vi "gettangentjob.vi"(0 "sample port":refnum<visa-resource-name>[](array[refnum]), 2 "sample sn":string[](array[string])) -> (6 "tangent":dbl[](array[numeric]), 7 "Array":bool[](array[boolean]))   [LabVIEW 2012]
uses:
  globalstatus.vi
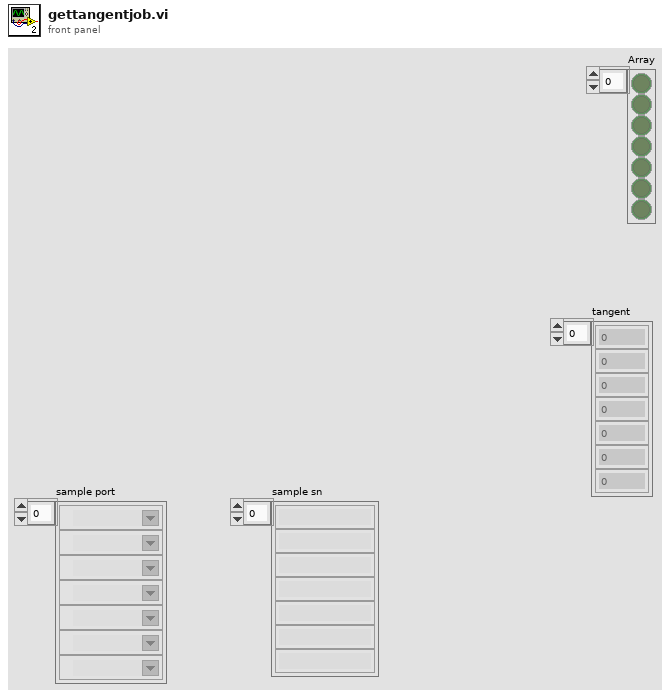
[diagram p1: front panel]
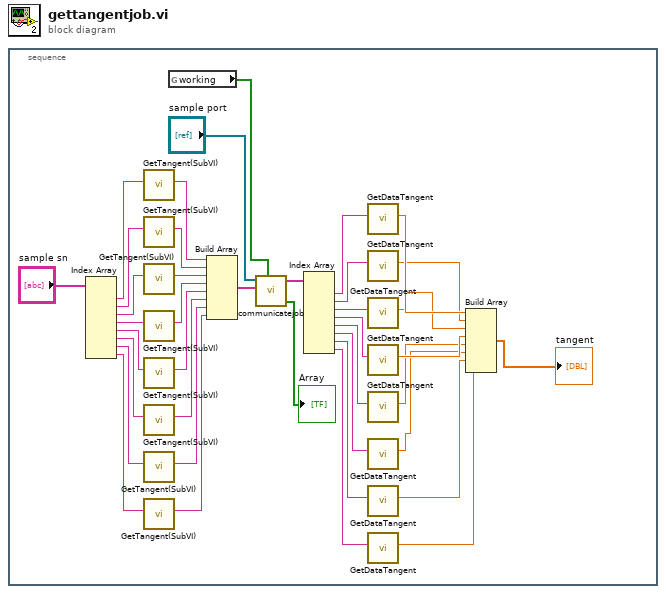
[diagram p0: block diagram]
diagram:
  n1 = stacked-sequence {
    frame #0 {
      n2 = Index Array(array="sample sn") -> (element #1=w38:string, element #2=w37:string, element #3=w36:string, element #4=w35:string, element #5=w34:string, element #6=w33:string, element #7=w32:string, element #8=w31:string)  [unwired: 8 in]
      n3 = call "GetTangent(SubVI).vi"("sn"=w38) -> ("output frame"=w28:string)  [unwired: 10 in]
      n4 = call "GetTangent(SubVI).vi"("sn"=w37) -> ("output frame"=w27:string)  [unwired: 10 in]
      n5 = call "GetTangent(SubVI).vi"("sn"=w36) -> ("output frame"=w26:string)  [unwired: 10 in]
      n6 = call "GetTangent(SubVI).vi"("sn"=w35) -> ("output frame"=w25:string)  [unwired: 10 in]
      n7 = call "GetTangent(SubVI).vi"("sn"=w34) -> ("output frame"=w24:string)  [unwired: 10 in]
      n8 = call "GetTangent(SubVI).vi"("sn"=w33) -> ("output frame"=w23:string)  [unwired: 10 in]
      n9 = call "GetTangent(SubVI).vi"("sn"=w32) -> ("output frame"=w22:string)  [unwired: 10 in]
      n10 = call "GetTangent(SubVI).vi"("sn"=w31) -> ("output frame"=w21:string)  [unwired: 10 in]
      n11 = global read "globalstatus.vi" "working"() -> (w29:bool[])
      n12 = Build Array(w28, w27, w26, w25, w24, w23, w22, w21) -> (w20:string[])
      n13 = call "communicatejob.vi"("sample port"="sample port", "condition"=w29, "send command"=w20) -> ("receive data"=w18:string[], "receive result"=→"Array":bool[])  [unwired: 2 in, 2 out]
      n14 = Index Array(array=w18) -> (element #1=w17:string, element #2=w16:string, element #3=w15:string, element #4=w14:string, element #5=w13:string, element #6=w12:string, element #7=w11:string, element #8=w10:string)  [unwired: 8 in]
      n15 = call "GetDataTangent.vi"("input data"=w17) -> ("tangent"=w9:dbl)  [unwired: 10 in]
      n16 = call "GetDataTangent.vi"("input data"=w16) -> ("tangent"=w8:dbl)  [unwired: 10 in]
      n17 = call "GetDataTangent.vi"("input data"=w15) -> ("tangent"=w7:dbl)  [unwired: 10 in]
      n18 = call "GetDataTangent.vi"("input data"=w14) -> ("tangent"=w6:dbl)  [unwired: 10 in]
      n19 = call "GetDataTangent.vi"("input data"=w13) -> ("tangent"=w5:dbl)  [unwired: 10 in]
      n20 = call "GetDataTangent.vi"("input data"=w12) -> ("tangent"=w4:dbl)  [unwired: 10 in]
      n21 = call "GetDataTangent.vi"("input data"=w11) -> ("tangent"=w3:dbl)  [unwired: 10 in]
      n22 = call "GetDataTangent.vi"("input data"=w10) -> ("tangent"=w2:dbl)  [unwired: 10 in]
      n23 = Build Array(w9, w8, w7, w6, w5, w4, w3, w2) -> (→"tangent":dbl[])
    }
  }
